vi "USB.vi"() -> ()   [LabVIEW 2018]
uses:
  <vilib>/myRIO/Common/Instrument Driver Framework/myRIO v1.0/UART/vis/myRIO v1.0 Close UART.vi
  <vilib>/myRIO/Common/Instrument Driver Framework/Utilities/vis/FPGA Ref Manager.vi
  <vilib>/myRIO/Common/Instrument Driver Framework/myRIO v1.0/myRIO v1.0 Reset FPGA.vi
  <vilib>/myRIO/Common/Instrument Driver Framework/myRIO v1.0/IRQ/vis/myRIO v1.0 IRQ Info FGV.vi
  <vilib>/myRIO/Common/Instrument Driver Framework/myRIO v1.0/IRQ/vis/myRIO v1.0 Timer IRQ Info FGV.vi
  <vilib>/myRIO/Common/Instrument Driver Framework/myRIO v1.0/IRQ/vis/myRIO v1.0 ISR Agent.vi
  <vilib>/myRIO/Instrument Drivers/Utilities/Utilities.lvlib
panel:
  out "length":i32
  in  "Stop (F)":bool
  out "Image Out":T1(plugin-control)
  in  "logfile base name":string="logfile"
  out "logfile name":path
  # "USB Flash Drive demo"
  # "1. Insert USB flash drive\n2. Enter logfile base name\n3. Run the VI\n4. Move NI myRIO to see onboard\n    accelerometer activity\n5. Stop the VI to save\n    acquired acceleration data to\n    logfile on USB flash drive"
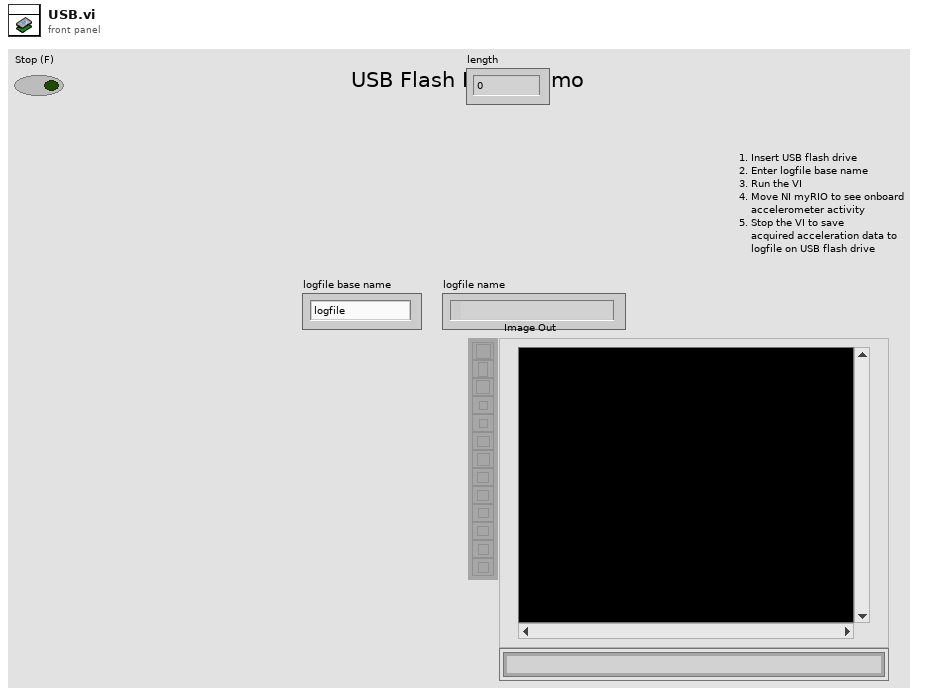
[diagram p1: front panel]
types:
  T1 = typedef "IMAQ Image.ctl" = refnum<image>
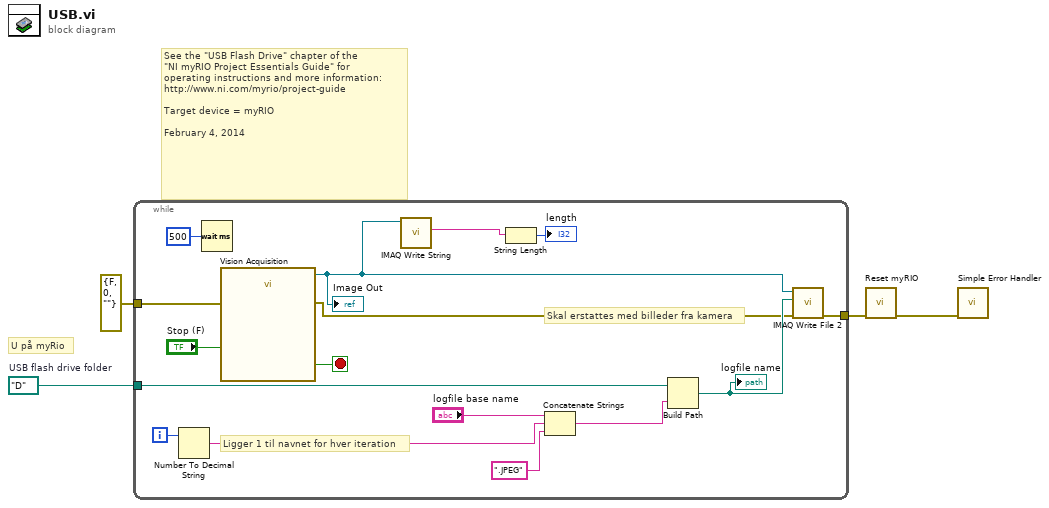
[diagram p0: block diagram]
diagram:
  w4 = path "D:/"  # USB flash drive folder
  # "U på myRio"
  # "See the \"USB Flash Drive\" chapter of the\n\"NI myRIO Project Essentials Guide\" for\noperating instructions and more information: \nhttp://www.ni.com/myrio/project-guide\n\nTarget device = myRIO\n\nFebruary 4, 2014"
  n1 = while {
    tunnel: w4 -> [w15]
    tunnel: errorcluster {"status"=FALSE, "code"=0, "source"=""} ("error in") -> [w9]
    tunnel: [w8] -> w2
    i -> [w13]
    stop <- w19 stop-if-true
    # "Ligger 1 til navnet for hver iteration"
    # "Skal erstattes med billeder fra kamera"
    n2 = Number To Decimal String(number=w13) -> (decimal integer string=w11:string)  [unwired: 1 in]
    n3 = Wait (ms)(milliseconds to wait=u32 500) -> ()  [unwired: 1 out]
    n4 = call "Vision Acquisition"("Stop (F)"="Stop (F)", "error in"=w9) -> ("Image Out"=w7:T1, "Stopped"=w19:bool, "error out"=w14:errorcluster)  [unwired: 23 in]
    "Image Out" <- w7
    n5 = call-poly "IMAQ Write String"("Image"=w7) -> ("File String Out"=w6:string)  [unwired: 8 in, 2 out]
    n6 = String Length(string=w6) -> (length=→"length":i32)
    n7 = Concatenate Strings "Concatenate Strings"("logfile base name", w11, ".JPEG" ("string")) -> (w16:string)
    n8 = Build Path(base path=w15, name or relative path=w16) -> (appended path=w17:path)
    "logfile name" <- w17
    n9 = call-poly "IMAQ Write File 2"("error in (no error)"=w14, "File Path"=w17, "Image"=w7) -> ("error out"=w8:errorcluster)  [unwired: 7 in, 1 out]
  }
  n10 = call <vilib>:"Reset myRIO.vi"("error in (no error)"=w2) -> ("error out"=w1:errorcluster)  [unwired: 10 in]
  n11 = call <vilib>:"Simple Error Handler.vi"("error in (no error)"=w1) -> ()  [unwired: 4 in, 5 out]
